vi "Wait Command SubVi.vi"(3 "GroupName":string, 4 "error in":errorcluster, 5 "reference in":refnum<k24>) -> (0 "Is Stop":bool, 1 "error out":errorcluster, 2 "reference out":refnum<k24>)   [LabVIEW 2017]
uses:
  Newport.XPS.CommandInterface
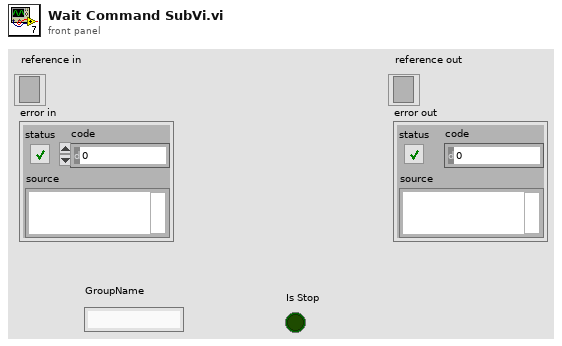
[diagram p1: front panel]
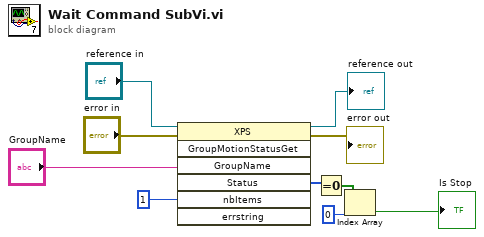
[diagram p0: block diagram]
diagram:
  n1 = invoke class="XPS" method="GroupMotionStatusGet"(reference="reference in", error in="error in", "GroupName"="GroupName", "nbItems"=1) -> (reference out=→"reference out":refnum<k24>, error out=→"error out":errorcluster, "Status"=w9:i32[])  [unwired: 3 in, 4 out]
  n2 = Equal To 0?(x=w9) -> (x = 0?=w8:bool[])
  n3 = Index Array(array=w8, index=0) -> (element=→"Is Stop":bool)
